vi "StopMod.vi"(8 "ErrorArray In":errorcluster[](array[cluster]), 10 "Module ID":i32=-1, 11 "Test.lvclass":refnum<class "Test.lvclass">) -> (0 "ErrorArray Out":errorcluster[](array[cluster]), 3 "Test.lvclass":refnum<class "Test.lvclass">)   [LabVIEW 2018, in "Test.lvclass"]
doc: "Stops all modules based on the Test Class information (Clone Registration, Module ID, and Module list)."
uses:
  Test.lvclass
  Test.lvclass/Test.ctl
  <userlib>/NIST/ModuleAdminLib/ModuleAdmin/ModuleAdmin.lvclass
  <userlib>/NIST/ModuleAdminLib/ModuleAdmin/ModuleAdmin.lvclass/ModuleAdmin.ctl
  <userlib>/NIST/ModuleAdminLib/ModuleAdmin/Accessors/Write CloneRegRef.vi
  Accessors/Write CloneReg.vi
  Accessors/Write ModuleIDs.vi
  Accessors/Write ModuleList.vi
  Accessors/Read CloneReg.vi
  Accessors/Read ModuleIDs.vi
  Accessors/Read ModuleList.vi
  <vilib>/Utility/error.llb/Error Cluster From Error Code.vi
  <userlib>/NIST/ModuleAdminLib/CloneRegistration/CloneRegistration.lvclass
  <vilib>/ErrorRing/Error Ring.xnode
  <userlib>/NIST/NISTErrorLib/NISTErrorLib.lvlib
  Sync/SyncModule/SyncModule.lvlib
  FGen/FgenModule/FgenModule.lvlib
  Analysis/AnalysisModule/AnalysisModule.lvlib
  Scope/ScopeModule/ScopeModule.lvlib
  AcPwr/AcPwrModule/AcPwrModule.lvlib
  Sensor/SensorShared/SensorShared.lvlib
  Digitizer/DigitizerShared/DigitizerShared.lvlib
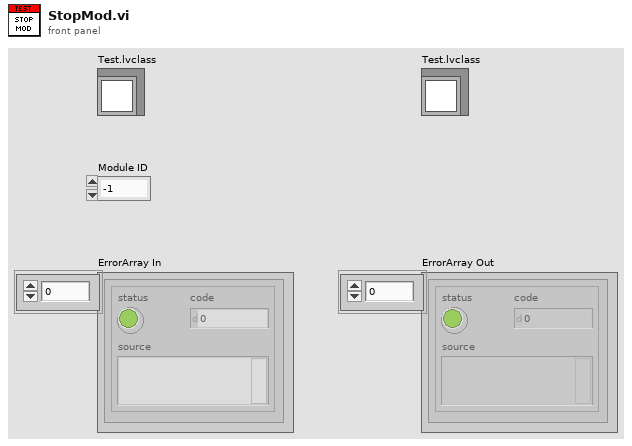
[diagram p1: front panel]
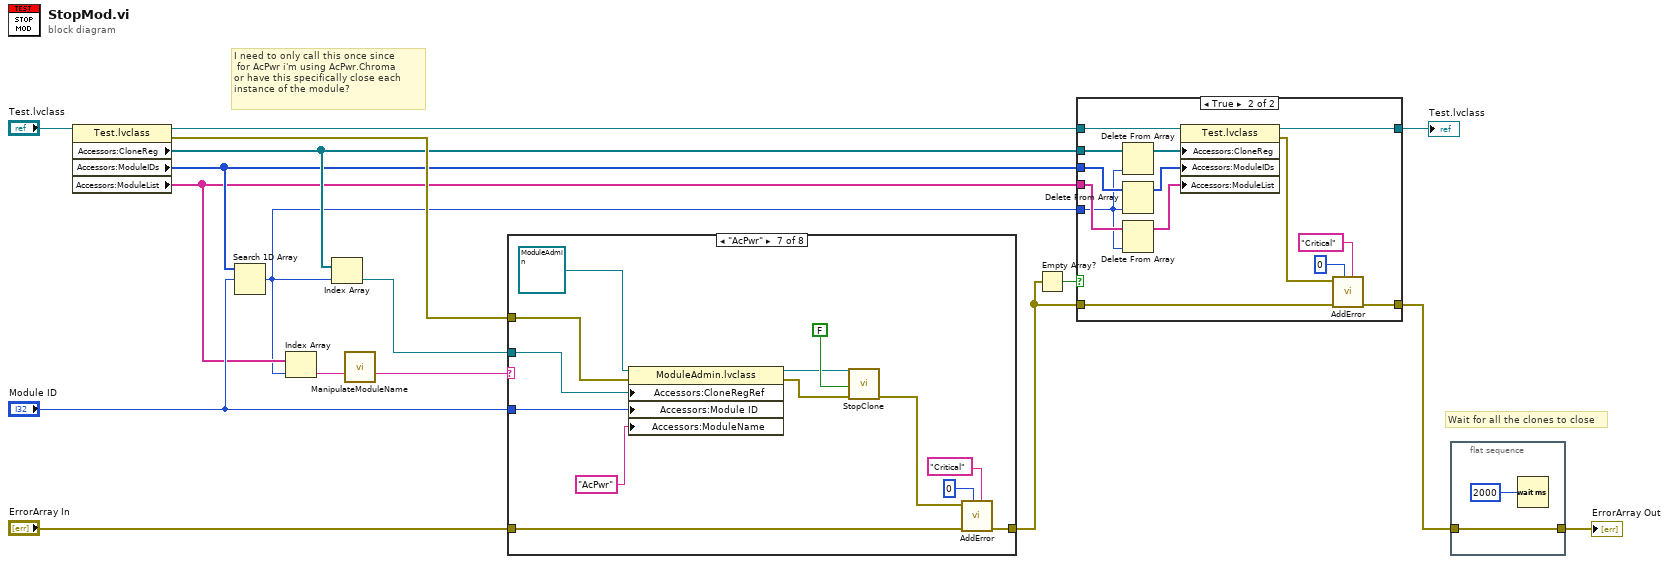
[diagram p0: block diagram]
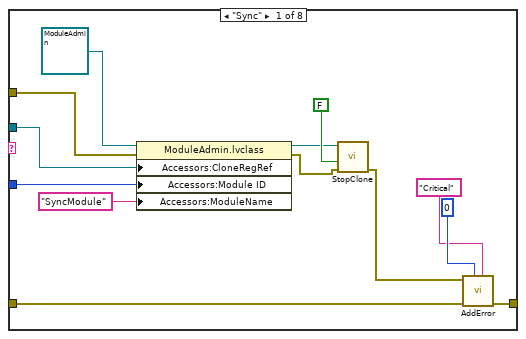
[diagram p3: hidden frame]
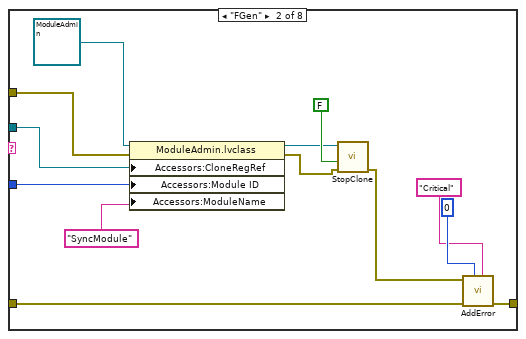
[diagram p4: hidden frame]
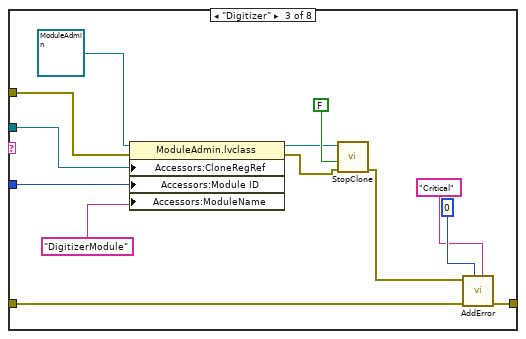
[diagram p5: hidden frame]
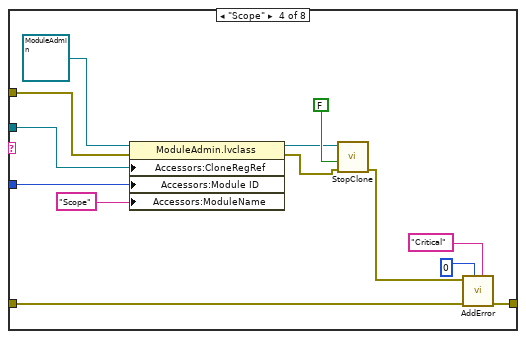
[diagram p6: hidden frame]
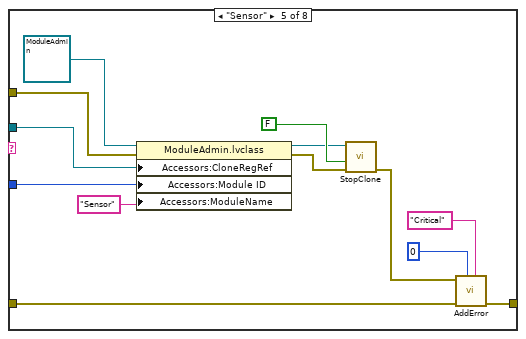
[diagram p7: hidden frame]
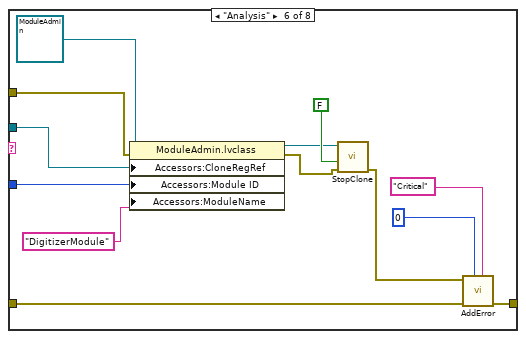
[diagram p8: hidden frame]
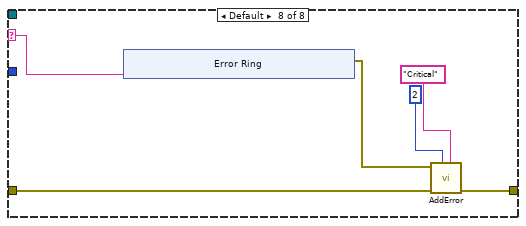
[diagram p9: hidden frame]
diagram:
  # "I need to only call this once since\n for AcPwr i'm using AcPwr.Chroma\nor have this specifically close each \ninstance of the module?"
  # "Wait for all the clones to close"
  n1 = property class="Test.lvclass"(reference="Test.lvclass") -> (reference out=w9:refnum<class "Test.lvclass">, error out=w16:errorcluster, "Accessors:CloneReg"=w7:refnum<data-value>[], "Accessors:ModuleIDs"=w6:i32[], "Accessors:ModuleList"=w5:string[])  [unwired: 1 in]
  n2 = Search 1D Array(1D array=w6, element="Module ID") -> (index of element=w3:i32)  [unwired: 1 in]
  n3 = Index Array(array=w5, index=w3) -> (element=w12:string)
  n4 = Index Array(array=w7, index=w3) -> (element=w10:refnum<data-value>)
  n5 = call "ManipulateModuleName.vi"("ModuleListSingleEntry"=w12) -> ("BeforeMatch:ModuleListSingleEntry"=w11:string)  [unwired: 9 in, 5 out]
  n6 = case shown="\"AcPwr\"" w11 {
    selector: w11 -> [_ _ _ _ _ _ _ w114]
    tunnel: "ErrorArray In" -> [w20 w33 w46 w59 w72 w85 w101 w110]
    tunnel: [w24 w37 w50 w63 w76 w89 w104 w109] -> w2
    tunnel: w10 -> [w29 w42 w55 w68 w81 w94 w107 _]
    tunnel: w16 -> [w18 w31 w44 w57 w71 w83 w96 _]
    tunnel: "Module ID" -> [w19 w32 w45 w58 w70 w84 w97 _]
    frame "Sync" {
      n7 = property class="ModuleAdmin.lvclass"(reference=refnum<class "ModuleAdmin.lvclass"> refnum ("ModuleAdmin.lvlib:ModuleAdmin.lvclass"), error in=w18, "Accessors:CloneRegRef"=w29, "Accessors:Module ID"=w19, "Accessors:ModuleName"="SyncModule" ("ModuleName")) -> (reference out=w26:refnum<class "ModuleAdmin.lvclass">, error out=w25:errorcluster)
      n8 = call "StopClone.vi"("error in (no error)"=w25, "Wait for Module to stop?"=FALSE, "ModuleAdmin"=w26) -> ("error out"=w21:errorcluster)  [unwired: 8 in]
      n9 = call <userlib>:"AddError.vi"("Severity"="Critical", "Priority"=u8 0, "ErrorArray In"=w20, "error in (no error)"=w21) -> ("ErrorArray Out"=w24:errorcluster[])  [unwired: 6 in, 1 out]
    }
    frame "FGen" {
      n10 = property class="ModuleAdmin.lvclass"(reference=refnum<class "ModuleAdmin.lvclass"> refnum ("ModuleAdmin.lvlib:ModuleAdmin.lvclass"), error in=w31, "Accessors:CloneRegRef"=w42, "Accessors:Module ID"=w32, "Accessors:ModuleName"="SyncModule" ("ModuleName")) -> (reference out=w39:refnum<class "ModuleAdmin.lvclass">, error out=w38:errorcluster)
      n11 = call "StopClone.vi"("error in (no error)"=w38, "Wait for Module to stop?"=FALSE, "ModuleAdmin"=w39) -> ("error out"=w34:errorcluster)  [unwired: 8 in]
      n12 = call <userlib>:"AddError.vi"("Severity"="Critical", "Priority"=u8 0, "ErrorArray In"=w33, "error in (no error)"=w34) -> ("ErrorArray Out"=w37:errorcluster[])  [unwired: 6 in, 1 out]
    }
    frame "Digitizer" {
      n13 = property class="ModuleAdmin.lvclass"(reference=refnum<class "ModuleAdmin.lvclass"> refnum ("ModuleAdmin.lvlib:ModuleAdmin.lvclass"), error in=w44, "Accessors:CloneRegRef"=w55, "Accessors:Module ID"=w45, "Accessors:ModuleName"="DigitizerModule" ("ModuleName")) -> (reference out=w52:refnum<class "ModuleAdmin.lvclass">, error out=w51:errorcluster)
      n14 = call "StopClone.vi"("error in (no error)"=w51, "Wait for Module to stop?"=FALSE, "ModuleAdmin"=w52) -> ("error out"=w47:errorcluster)  [unwired: 8 in]
      n15 = call <userlib>:"AddError.vi"("Severity"="Critical", "Priority"=u8 0, "ErrorArray In"=w46, "error in (no error)"=w47) -> ("ErrorArray Out"=w50:errorcluster[])  [unwired: 6 in, 1 out]
    }
    frame "Scope" {
      n16 = property class="ModuleAdmin.lvclass"(reference=refnum<class "ModuleAdmin.lvclass"> refnum ("ModuleAdmin.lvlib:ModuleAdmin.lvclass"), error in=w57, "Accessors:CloneRegRef"=w68, "Accessors:Module ID"=w58, "Accessors:ModuleName"="Scope" ("ModuleName")) -> (reference out=w65:refnum<class "ModuleAdmin.lvclass">, error out=w64:errorcluster)
      n17 = call "StopClone.vi"("error in (no error)"=w64, "Wait for Module to stop?"=FALSE, "ModuleAdmin"=w65) -> ("error out"=w60:errorcluster)  [unwired: 8 in]
      n18 = call <userlib>:"AddError.vi"("Severity"="Critical", "Priority"=u8 0, "ErrorArray In"=w59, "error in (no error)"=w60) -> ("ErrorArray Out"=w63:errorcluster[])  [unwired: 6 in, 1 out]
    }
    frame "Sensor" {
      n19 = property class="ModuleAdmin.lvclass"(reference=refnum<class "ModuleAdmin.lvclass"> refnum ("ModuleAdmin.lvlib:ModuleAdmin.lvclass"), error in=w71, "Accessors:CloneRegRef"=w81, "Accessors:Module ID"=w70, "Accessors:ModuleName"="Sensor" ("ModuleName")) -> (reference out=w78:refnum<class "ModuleAdmin.lvclass">, error out=w77:errorcluster)
      n20 = call "StopClone.vi"("error in (no error)"=w77, "Wait for Module to stop?"=FALSE, "ModuleAdmin"=w78) -> ("error out"=w73:errorcluster)  [unwired: 8 in]
      n21 = call <userlib>:"AddError.vi"("Severity"="Critical", "Priority"=u8 0, "ErrorArray In"=w72, "error in (no error)"=w73) -> ("ErrorArray Out"=w76:errorcluster[])  [unwired: 6 in, 1 out]
    }
    frame "Analysis" {
      n22 = property class="ModuleAdmin.lvclass"(reference=refnum<class "ModuleAdmin.lvclass"> refnum ("ModuleAdmin.lvlib:ModuleAdmin.lvclass"), error in=w83, "Accessors:CloneRegRef"=w94, "Accessors:Module ID"=w84, "Accessors:ModuleName"="DigitizerModule" ("ModuleName")) -> (reference out=w91:refnum<class "ModuleAdmin.lvclass">, error out=w90:errorcluster)
      n23 = call "StopClone.vi"("error in (no error)"=w90, "Wait for Module to stop?"=FALSE, "ModuleAdmin"=w91) -> ("error out"=w86:errorcluster)  [unwired: 8 in]
      n24 = call <userlib>:"AddError.vi"("Severity"="Critical", "Priority"=u8 0, "ErrorArray In"=w85, "error in (no error)"=w86) -> ("ErrorArray Out"=w89:errorcluster[])  [unwired: 6 in, 1 out]
    }
    frame "AcPwr" {
      n25 = property class="ModuleAdmin.lvclass"(reference=refnum<class "ModuleAdmin.lvclass"> refnum ("ModuleAdmin.lvlib:ModuleAdmin.lvclass"), error in=w96, "Accessors:CloneRegRef"=w107, "Accessors:Module ID"=w97, "Accessors:ModuleName"="AcPwr" ("ModuleName")) -> (reference out=w98:refnum<class "ModuleAdmin.lvclass">, error out=w105:errorcluster)
      n26 = call "StopClone.vi"("error in (no error)"=w105, "Wait for Module to stop?"=FALSE, "ModuleAdmin"=w98) -> ("error out"=w100:errorcluster)  [unwired: 8 in]
      n27 = call <userlib>:"AddError.vi"("Severity"="Critical", "Priority"=u8 0, "ErrorArray In"=w101, "error in (no error)"=w100) -> ("ErrorArray Out"=w104:errorcluster[])  [unwired: 6 in, 1 out]
    }
    frame Default {
      n28 = xnode "Error Ring"("parameter 0"=w114) -> ("error out"=w111:errorcluster)
      n29 = call <userlib>:"AddError.vi"("Severity"="Critical", "Priority"=u8 2, "ErrorArray In"=w110, "error in (no error)"=w111) -> ("ErrorArray Out"=w109:errorcluster[])  [unwired: 6 in, 1 out]
    }
  }
  n30 = Empty Array?(array=w2) -> (empty?=w8:bool)
  n31 = case shown="True" w8 {
    tunnel: w9 -> [w123 w137]
    tunnel: w7 -> [_ w135]
    tunnel: w6 -> [_ w134]
    tunnel: w5 -> [_ w133]
    tunnel: [w123 w136] -> w4
    tunnel: w3 -> [_ w132]
    tunnel: w2 -> [w122 w125]
    tunnel: [w122 w124] -> w1
    frame False {
    }
    frame True {
      n32 = Delete From Array(array=w135, index=w132) -> (array with subset deleted=w131:refnum<data-value>[])  [unwired: 1 in, 1 out]
      n33 = Delete From Array(array=w134, index=w132) -> (array with subset deleted=w130:i32[])  [unwired: 1 in, 1 out]
      n34 = Delete From Array(array=w133, index=w132) -> (array with subset deleted=w129:string[])  [unwired: 1 in, 1 out]
      n35 = property class="Test.lvclass"(reference=w137, "Accessors:CloneReg"=w131, "Accessors:ModuleIDs"=w130, "Accessors:ModuleList"=w129) -> (reference out=w136:refnum<class "Test.lvclass">, error out=w126:errorcluster)  [unwired: 1 in]
      n36 = call <userlib>:"AddError.vi"("Severity"="Critical", "Priority"=u8 0, "ErrorArray In"=w125, "error in (no error)"=w126) -> ("ErrorArray Out"=w124:errorcluster[])  [unwired: 6 in, 1 out]
    }
  }
  "Test.lvclass" <- w4
  n37 = flat-sequence {
    tunnel: [w139] -> w15
    tunnel: w1 -> [w139]
    frame #0 {
      n38 = Wait (ms)(milliseconds to wait=u32 2000) -> ()  [unwired: 1 out]
    }
  }
  "ErrorArray Out" <- w15
